vi "X_C_2500_5.vi"(0 "ek":dbl format="%#_13g", 2 "length":i32=5, 3 "q":dbl[](array[numeric])=[1.0, 1.0, 1.0, 1.0, 1.0] format="%#_13g") -> (5 "uk":dbl format="%#_13g")   [LabVIEW 2015]
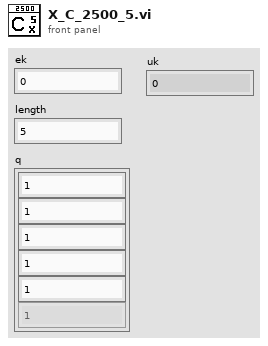
[diagram p1: front panel]
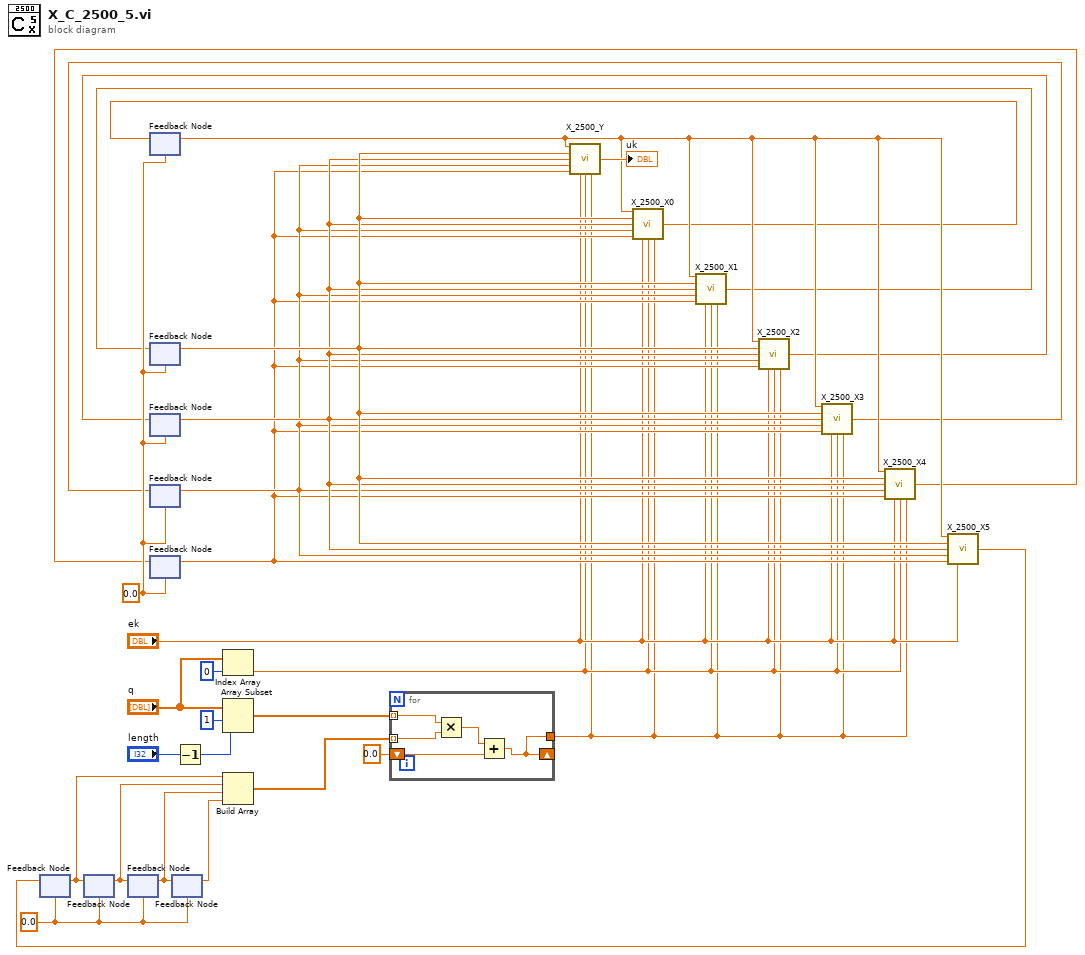
[diagram p0: block diagram]
diagram:
  w17 = 0.0
  w22 = 0.0
  n1 = feedback #1(w17) -> (w18:dbl)
  n2 = feedback #2(w17) -> (w19:dbl)
  n3 = feedback-in #2(w18) -> ()
  n4 = feedback #3(w17) -> (w20:dbl)
  n5 = feedback-in #3(w19) -> ()
  n6 = feedback #4(w22) -> (w14:dbl)
  n7 = feedback #5(w22) -> (w13:dbl)
  n8 = feedback #6(w22) -> (w12:dbl)
  n9 = feedback #7(w22) -> (w11:dbl)
  n10 = feedback #8(w22) -> (w10:dbl)
  n11 = feedback #9(w17) -> (w21:dbl)
  n12 = feedback-in #9(w20) -> ()
  n13 = Decrement(x="length") -> (x-1=w23:i32)
  n14 = Index Array(array="q", index=0) -> (element=w3:dbl)
  n15 = Array Subset(array="q", index=1, length=w23) -> (w24:dbl[])
  n16 = Build Array(w18, w19, w20, w21) -> (w16:dbl[])
  n17 = for {
    tunnel: w16 -> [w33] mode=indexing
    tunnel: w24 -> [w34] mode=indexing
    shift-right: [w30] -> _
    shift-left: 0.0 -> [w31]
    tunnel: [w30] -> w2
    n18 = Multiply(x=w34, y=w33) -> (x*y=w32:dbl)
    n19 = Add(x=w32, y=w31) -> (x+y=w30:dbl)
  }
  n20 = call "X_2500_Y.vi"("x0"=w14, "x1"=w13, "x2"=w12, "x3"=w11, "x4"=w10, "e"="ek", "q0"=w3, "qzsum"=w2) -> ("Yout"=→"uk":dbl)  [unwired: 7 in]
  n21 = call "X_2500_X0.vi"("x0"=w14, "x1"=w13, "x2"=w12, "x3"=w11, "x4"=w10, "e"="ek", "q0"=w3, "qzsum"=w2) -> ("X0out"=w9:dbl)  [unwired: 7 in]
  n22 = feedback-in #4(w9) -> ()
  n23 = call "X_2500_X1.vi"("x0"=w14, "x1"=w13, "x2"=w12, "x3"=w11, "x4"=w10, "e"="ek", "q0"=w3, "qzsum"=w2) -> ("X1out"=w8:dbl)  [unwired: 7 in]
  n24 = feedback-in #5(w8) -> ()
  n25 = call "X_2500_X2.vi"("x0"=w14, "x1"=w13, "x2"=w12, "x3"=w11, "x4"=w10, "e"="ek", "q0"=w3, "qzsum"=w2) -> ("X2out"=w7:dbl)  [unwired: 7 in]
  n26 = feedback-in #6(w7) -> ()
  n27 = call "X_2500_X3.vi"("x0"=w14, "x1"=w13, "x2"=w12, "x3"=w11, "x4"=w10, "e"="ek", "q0"=w3, "qzsum"=w2) -> ("X3out"=w6:dbl)  [unwired: 7 in]
  n28 = feedback-in #7(w6) -> ()
  n29 = call "X_2500_X4.vi"("x0"=w14, "x1"=w13, "x2"=w12, "x3"=w11, "x4"=w10, "e"="ek", "q0"=w3, "qzsum"=w2) -> ("X4out"=w5:dbl)  [unwired: 7 in]
  n30 = feedback-in #8(w5) -> ()
  n31 = call "X_2500_X5.vi"("x0"=w14, "x1"=w13, "x2"=w12, "x3"=w11, "x4"=w10, "e"="ek") -> ("X5out"=w1:dbl)  [unwired: 9 in]
  n32 = feedback-in #1(w1) -> ()
